vi "set_PFI_line.vi"(10 "out":tag="Dev1/port2/line2", 11 "ON/OFF":bool) -> ()   [LabVIEW 2021]
uses:
  <vilib>/DAQmx/write.llb/DAQmx Write (Digital Bool 1Line 1Point).vi
  <vilib>/DAQmx/create/channels.llb/DAQmx Create Channel (DO-Digital Output).vi
  <vilib>/DAQmx/miscellaneous.llb/DAQmx Fill In Error Info.vi
panel:
  # "Port 2, lines 1,2,3,4 (not 0)"
  # "Ch 6"
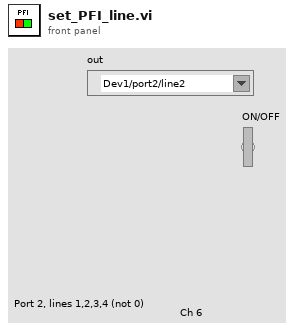
[diagram p1: front panel]
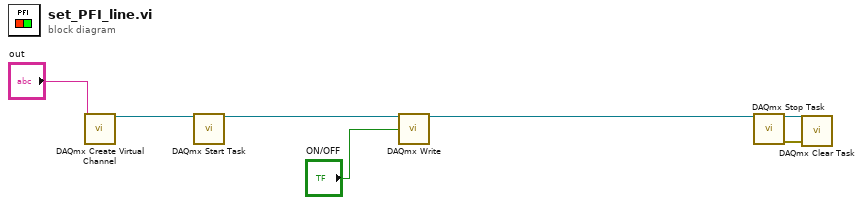
[diagram p0: block diagram]
diagram:
  n1 = call-poly <vilib>:"DAQmx Create Virtual Channel.vi"("lines"="out") -> ("task out"=w5:refnum<k21>)  [unwired: 13 in, 1 out]
  n2 = call <vilib>:"DAQmx Start Task.vi"("task/channels in"=w5) -> ("task out"=w3:refnum<k21>)  [unwired: 13 in, 1 out]
  n3 = call-poly <vilib>:"DAQmx Write.vi"("task/channels in"=w3, "data"="ON/OFF") -> ("task out"=w2:refnum<k21>)  [unwired: 11 in, 2 out]
  n4 = call <vilib>:"DAQmx Stop Task.vi"("task/channels in"=w2) -> ("task out"=w7:refnum<k21>, "error out"=w6:errorcluster)  [unwired: 13 in]
  n5 = call <vilib>:"DAQmx Clear Task.vi"("task in"=w7, "error in"=w6) -> ()  [unwired: 13 in, 1 out]
